vi "Configure Math Function.vi"(7 "Math Reference Method (0: Percent)":u16(ring) items=["Percent", "Input"], 8 "error in (no error)":errorcluster, 9 "Enable Math Function (T:Enable)":bool=TRUE, 10 "Percent Reference (1)":dbl=1.0 min=-100000000.0 max=100000000.0 format="%#.3f", 11 "VISA resource name":refnum<visa-resource-name>) -> (0 "error out":errorcluster, 3 "VISA resource name out":refnum<visa-resource-name>)   [LabVIEW 2021, in "BK Precision 5491B.lvlib"]
doc: "Configures and enables the math function.\n\n<b>Note: Math function can only be applied to the primary measurement function.</b>"
uses:
  <instrlib>/BK Precision 5491B/BK Precision 5491B.lvlib
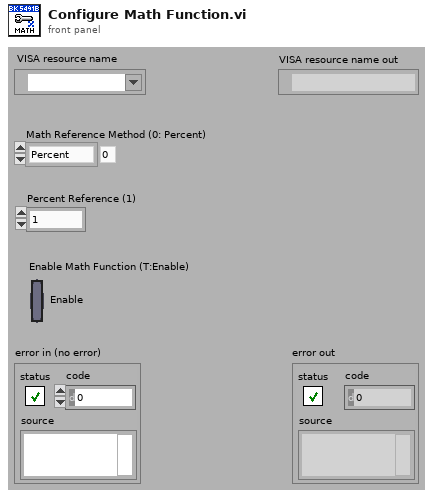
[diagram p1: front panel]
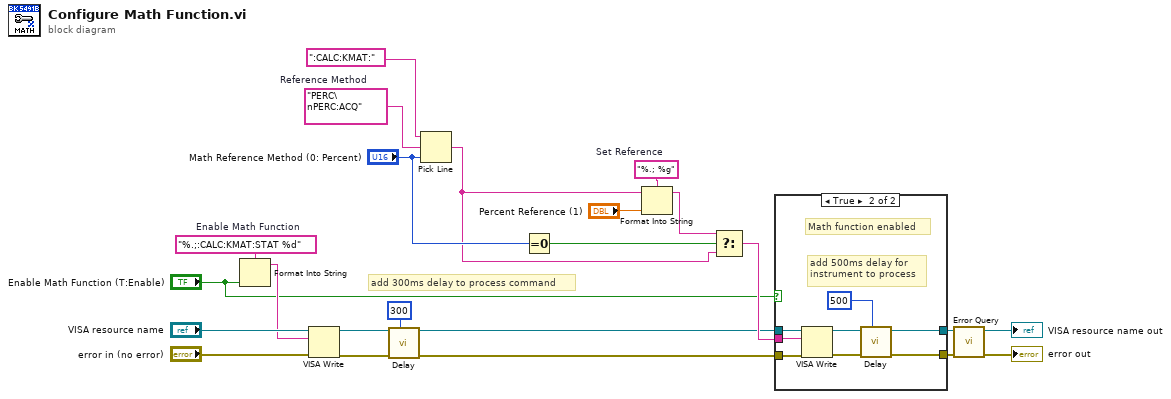
[diagram p0: block diagram]
diagram:
  w11 = "%.;:CALC:KMAT:STAT %d"  # Enable Math Function
  w20 = "%.; %g"  # Set Reference
  w21 = "PERC\nPERC:ACQ"  # Reference Method
  # "add 300ms delay to process command"
  n1 = Format Into String(format string=w11, "Enable Math Function (T:Enable)") -> (resulting string=w8:string)  [unwired: 2 in, 1 out]
  n2 = VISA Write(VISA resource name="VISA resource name", write buffer=w8, error in (no error)="error in (no error)") -> (VISA resource name out=w6:refnum<visa-resource-name>, error out=w5:errorcluster)  [unwired: 1 out]
  n3 = call <instrlib>:"Delay.vi"("Delay Time (0)"=u32 300, "error in (no error)"=w5, "VISA resource name"=w6) -> ("error out"=w4:errorcluster, "VISA resource name out"=w3:refnum<visa-resource-name>)  [unwired: 7 in]
  n4 = Pick Line(string ("")=":CALC:KMAT:", multi-line string=w21, line index="Math Reference Method (0: Percent)") -> (output string=w12:string)
  n5 = Equal To 0?(x="Math Reference Method (0: Percent)") -> (x = 0?=w15:bool)
  n6 = Format Into String(format string=w20, initial string=w12, "Percent Reference (1)") -> (resulting string=w13:string)  [unwired: 1 in, 1 out]
  n7 = Select(t=w13, s=w15, f=w12) -> (s? t:f=w7:string)
  n8 = case shown="True" "Enable Math Function (T:Enable)" {
    tunnel: [w25 w32] -> w19
    tunnel: [w24 w31] -> w18
    tunnel: w7 -> [_ w28]
    tunnel: w4 -> [w24 w27]
    tunnel: w3 -> [w25 w26]
    frame False {
      # "Math function disabled"
    }
    frame True {
      # "Math function enabled"
      # "add 500ms delay for\ninstrument to process"
      n9 = VISA Write(VISA resource name=w26, write buffer=w28, error in (no error)=w27) -> (VISA resource name out=w33:refnum<visa-resource-name>, error out=w30:errorcluster)  [unwired: 1 out]
      n10 = call <instrlib>:"Delay.vi"("Delay Time (0)"=u32 500, "error in (no error)"=w30, "VISA resource name"=w33) -> ("error out"=w31:errorcluster, "VISA resource name out"=w32:refnum<visa-resource-name>)  [unwired: 7 in]
    }
  }
  n11 = call <instrlib>:"Error Query.vi"("error in (no error)"=w18, "VISA resource name"=w19) -> ("error out"=→"error out":errorcluster, "VISA resource name out"=→"VISA resource name out":refnum<visa-resource-name>)  [unwired: 7 in, 1 out]
